vi "Write Bounds Prefs.vi"(8 "error in (no error)":errorcluster, 11 "PluginGUI in":refnum<class "PluginGUI.lvclass">) -> (0 "error out":errorcluster, 3 "PluginGUI out":refnum<class "PluginGUI.lvclass">)   [LabVIEW 2020, in "VolatusGUI.lvlib" / "PluginGUI.lvclass"]
uses:
  PluginGUI.lvclass
  PluginGUI.lvclass/PluginGUI.ctl
  Volatus/MessageQ/MessageQ.lvclass/MessageQ.ctl
  GUI Helper/GUI Helper.lvclass
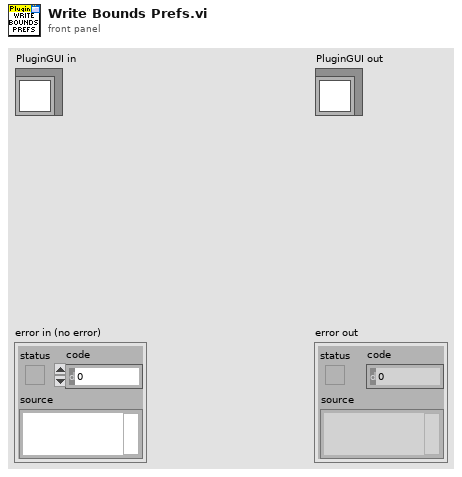
[diagram p1: front panel]
types:
  T1 = typedef "LVRectTypeDef.ctl" = cluster{"Left":i16, "Top":i16, "Right":i16, "Bottom":i16}
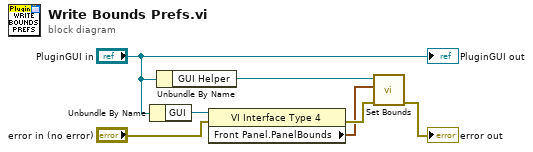
[diagram p0: block diagram]
diagram:
  n1 = Unbundle By Name("PluginGUI in") -> ("GUI"=w6:refnum<vi>)
  n2 = Unbundle By Name("PluginGUI in") -> ("GUI Helper"=w3:refnum<class "MessageQ.lvclass">)
  n3 = property class="VI Interface Type 4"(reference=w6, error in="error in (no error)") -> (error out=w7:errorcluster, "Front Panel.PanelBounds"=w2:T1)  [unwired: 1 out]
  n4 = call "Set Bounds.vi"("error in (no error)"=w7, "Bounds"=w2, "GUI Helper in"=w3) -> ("error out"=→"error out":errorcluster)  [unwired: 7 in, 1 out]
  "PluginGUI out" <- "PluginGUI in"
